vi "Publish Sample.vi"(8 "error in (no error)":errorcluster, 9 "Sample":refnum<class "Sample.lvclass">, 11 "Preparation Line in":refnum<class "Preparation Line.lvclass">) -> (0 "error out":errorcluster, 3 "Preparation Line out":refnum<class "Preparation Line.lvclass">)   [LabVIEW 2015, in "cRIO-Carbondioxide.lvlib" / "CO2-Actor.lvlib" / "Preparation Line.lvclass"]
uses:
  Preparation Line.lvclass
  subs/Sample/Sample.lvclass
  Preparation Line.lvclass/Preparation Line.ctl
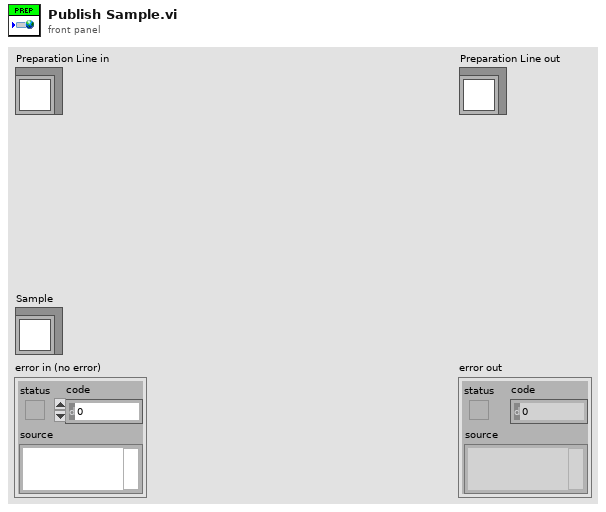
[diagram p1: front panel]
types:
  T1 = typedef "Sample Container.ctl" = cluster{"Sample In":refnum<k21>, "Sample Name":refnum<k21>, "Ti Cathode":refnum<k21>, "SampleQ":refnum<queue>}
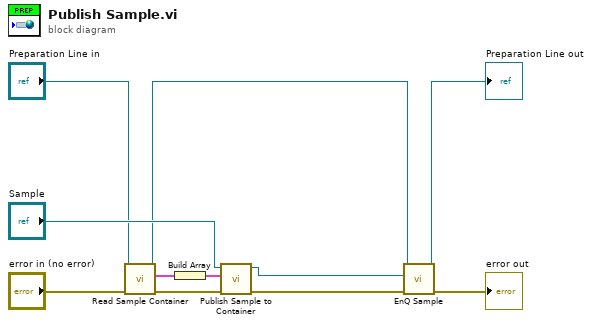
[diagram p0: block diagram]
diagram:
  n1 = call "Read Sample Container.vi"("error in (no error)"="error in (no error)", "Preparation Line in"="Preparation Line in") -> ("error out"=w9:errorcluster, "Container"=w7:T1, "Preparation Line out"=w3:refnum<class "Preparation Line.lvclass">)  [unwired: 6 in, 1 out]
  n2 = Build Array(w7) -> (w6:T1[])
  n3 = call "Publish Sample to Container.vi"("error in (no error)"=w9, "Containers"=w6, "Sample in"="Sample") -> ("error out"=w5:errorcluster, "Sample out"=w1:refnum<class "Sample.lvclass">)  [unwired: 7 in]
  n4 = call "EnQ Sample.vi"("error in (no error)"=w5, "Sample.lvclass"=w1, "Preparation Line in"=w3) -> ("error out"=→"error out":errorcluster, "Preparation Line out"=→"Preparation Line out":refnum<class "Preparation Line.lvclass">)  [unwired: 7 in]
